vi "GE 5565PIORC.PIO.Window.Size.vi"(8 "error in (no error)":errorcluster, 11 "GE 5565PIORC in":refnum<class "GE 5565PIORC.lvclass">) -> (0 "error out":errorcluster, 2 "window size":u32 format="%.0pB", 3 "GE 5565PIORC out":refnum<class "GE 5565PIORC.lvclass">)   [LabVIEW 2016, in "GE 5565PIORC.lvclass"]
doc: "Returns the configured <B>window size</B> of the PIO Window by computing the two's compliment of the PIO Local Mask. This window size is determined by the S1 DIP switches on the GE 5565PIORC board, and is read-only."
uses:
  GE 5565PIORC.lvclass
  GE 5565PIORC.lvclass/GE 5565PIORC.ctl
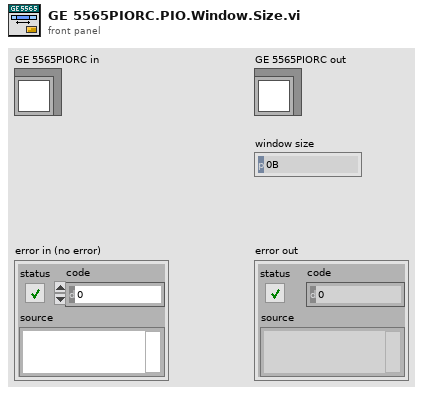
[diagram p1: front panel]
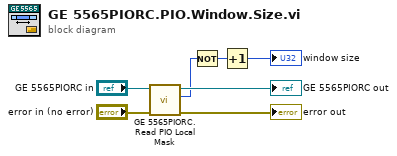
[diagram p0: block diagram]
diagram:
  n1 = call "GE 5565PIORC.Read PIO Local Mask.vi"("error in (no error)"="error in (no error)", "GE 5565PIORC in"="GE 5565PIORC in") -> ("error out"=→"error out":errorcluster, "PIO Local Mask"=w2:u32, "GE 5565PIORC out"=→"GE 5565PIORC out":refnum<class "GE 5565PIORC.lvclass">)  [unwired: 7 in]
  n2 = Not(x=w2) -> (.not. x?=w3:u32)
  n3 = Increment(x=w3) -> (x+1=→"window size":u32)
